vi "Uninit.vi"(11 "Queue Msg Type Strategy in":refnum<class "Queue Msg Type Strategy.lvclass">) -> (0 "error out":errorcluster)   [LabVIEW 2021, in "jettl.lvlib" / "Msg Type Strategy.lvlib" / "Queue Msg Type Strategy.lvclass"]
uses:
  Queue Msg Type Strategy.lvclass
  Queue Msg Type Strategy.lvclass/Queue Msg Type Strategy.ctl
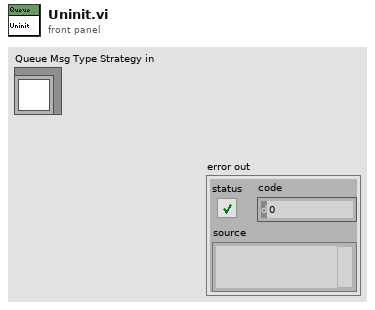
[diagram p1: front panel]
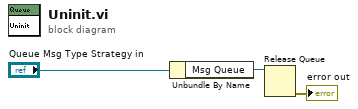
[diagram p0: block diagram]
diagram:
  n1 = Unbundle By Name("Queue Msg Type Strategy in") -> ("Msg Queue"=w1:refnum<queue>)
  n2 = Release Queue(queue=w1) -> (error out=→"error out":errorcluster)  [unwired: 2 in, 2 out]
